vi "Render Matrix.vi"(6 "origin":cluster{"x":i16, "y":i16}={"x"=10, "y"=10}, 7 "format string":string=" %#g", 10 "A":dbl[][](array[numeric])=[[2.0, 0.0, 0.01], [0.0, 2.0, 0.0012], [2222.0, 12.0, 212.0]] format="%.2f", 11 "picture in":picture) -> (3 "picture out":picture)   [LabVIEW 2013]
uses:
  <vilib>/addons/Control Design/_Utility/NI_LinSys_Rendering.lvlib
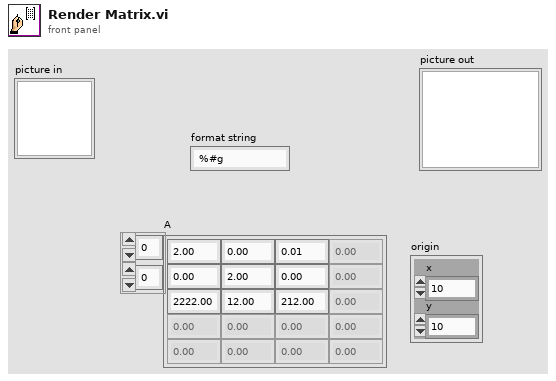
[diagram p1: front panel]
types:
  T1 = enum16{"User-specified Font", "Application Font", "System Font", "Dialog Font"}
  T2 = cluster{"Font Name:":string, "Size":i16, "Strikeout?":bool, "Italic?":bool, "Underline?":bool, "Outline?":bool, "Shadow?":bool, "Bold?":bool}
  T3 = cluster{"Origins Position":cluster{"x":i16, "y":i16}[][], "Left Bracket":cluster{"x":i16, "y":u32}[], "Right Bracket":cluster{"x":u32, "y":u32}[]}
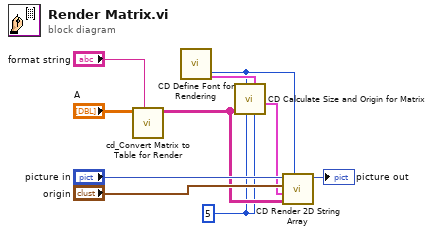
[diagram p0: block diagram]
diagram:
  w1 = u32 5 ("Width Gap")
  n1 = call <vilib>:"cd_Convert Matrix to Table for Render.vi"("format string"="format string", "A"="A") -> ("Matrix A 2"=w5:string[][])  [unwired: 9 in]
  n2 = call <vilib>:"CD Define Font for Rendering.vi"() -> ("matrix desired font(Application) 2"=w7:T1, "Matrix Number"=w8:T2)  [unwired: 9 in, 5 out]
  n3 = call <vilib>:"CD Calculate Size and Origin for Matrix.vi"("Height Gap"=w1, "[user-specified font]"=w8, "Width Gap"=w1, "desired font(Application)"=w7, "Matrix A"=w5) -> ("output cluster"=w4:T3)  [unwired: 5 in, 1 out]
  n4 = call <vilib>:"CD Render 2D String Array.vi"("desired font(Application)"=w7, "Matrix"=w5, "output cluster"=w4, "origin"="origin", "picture in"="picture in") -> ("picture out"=→"picture out":picture)  [unwired: 6 in]
